vi "Get Coverage for VIs in Project.vi"(8 "error in (no error)":errorcluster, 10 "Project Path":path, 11 "Coverage Analyzer in":refnum<class "Coverage Analyzer.lvclass">) -> (0 "error out":errorcluster, 2 "Code Coverage":map{path, dbl}(c390), 3 "Coverage Analyzer out":refnum<class "Coverage Analyzer.lvclass">)   [LabVIEW 2020, in "Coverage Analyzer.lvclass"]
uses:
  Coverage Analyzer.lvclass
  Coverage Analyzer.lvclass/Coverage Analyzer.ctl
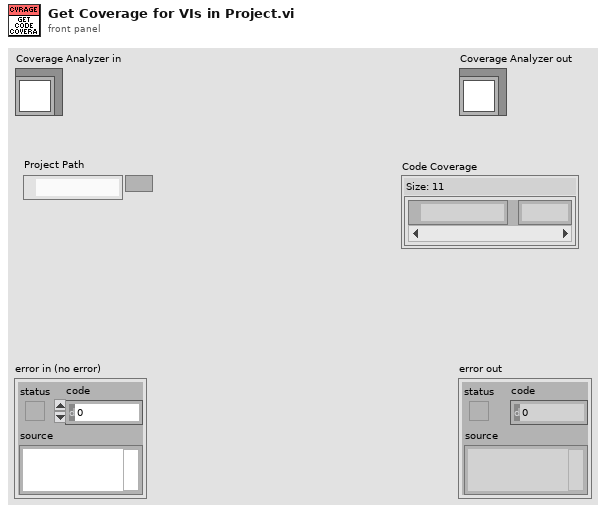
[diagram p1: front panel]
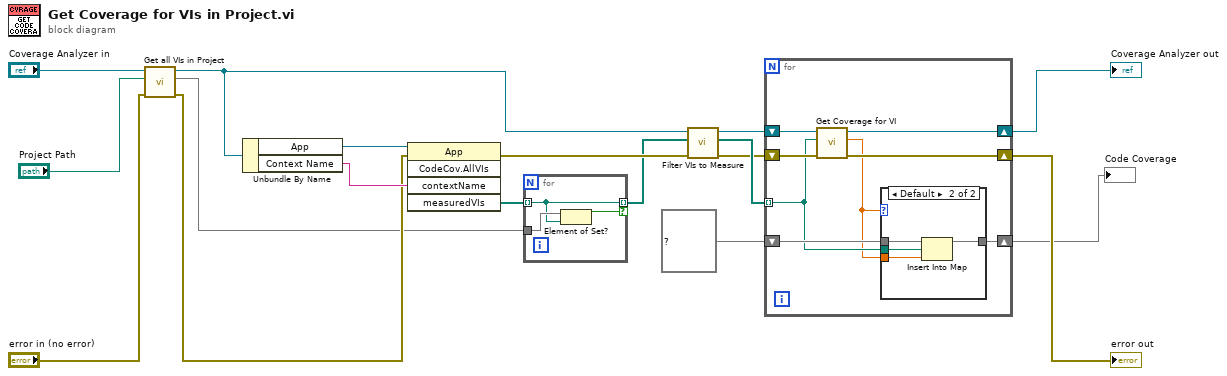
[diagram p0: block diagram]
diagram:
  n1 = call "Get all VIs in Project.vi"("error in (no error)"="error in (no error)", "Path"="Project Path", "Coverage Analyzer in"="Coverage Analyzer in") -> ("error out"=w4:errorcluster, "VIs"=w3:set{path}, "Coverage Analyzer out"=w7:refnum<class "Coverage Analyzer.lvclass">)  [unwired: 6 in]
  n2 = Unbundle By Name(w7) -> ("App"=w17:refnum<vi>, "Context Name"=w18:string)
  n3 = invoke class="App" method="CodeCov.AllVIs"(reference=w17, error in=w4, "contextName"=w18) -> (error out=w10:errorcluster, "measuredVIs"=w2:path[])  [unwired: 2 in, 3 out]
  n4 = for {
    tunnel: w3 -> [w21]
    tunnel: w2 -> [w20] mode=indexing
    tunnel: [w20] -> w1 mode=indexing if=w19
    n5 = Element of Set?(10:w20, 11:w21) -> (3:w19:bool)
  }
  n6 = call "Filter VIs to Measure.vi"("error in (no error)"=w10, "VI Paths"=w1, "Coverage Analyzer in"=w7) -> ("error out"=w9:errorcluster, "Filtered VI Paths"=w11:path[], "Coverage Analyzer out"=w12:refnum<class "Coverage Analyzer.lvclass">)  [unwired: 6 in]
  n7 = for {
    shift-right: [w28] -> w16
    shift-left: w12 -> [w29]
    shift-right: [w26] -> w15
    shift-left: w9 -> [w27]
    tunnel: w11 -> [w23] mode=indexing
    shift-right: [w24] -> w13
    shift-left: map{path, dbl} {} ("Code Coverage") -> [w25]
    n8 = call "Get Coverage for VI.vi"("error in (no error)"=w27, "VI Path"=w23, "Coverage Analyzer in"=w29) -> ("error out"=w26:errorcluster, "Percentage"=w22:dbl, "Coverage Analyzer out"=w28:refnum<class "Coverage Analyzer.lvclass">)  [unwired: 5 in, 1 out]
    n9 = case shown="Default" w22 {
      tunnel: w25 -> [w30 w34]
      tunnel: [w30 w33] -> w24
      tunnel: w22 -> [_ w32]
      tunnel: w23 -> [_ w31]
      frame 0 {
      }
      frame Default {
        n10 = Insert Into Map(map in=w34, key=w31, value=w32) -> (map out=w33:map{path, dbl})  [unwired: 2 out]
      }
    }
  }
  "error out" <- w15
  "Coverage Analyzer out" <- w16
  "Code Coverage" <- w13
